vi "Laser-Repetition.vi"(2 "error in (no error)":errorcluster, 5 "VISA resource name":refnum<visa-resource-name>) -> (0 "error out":errorcluster, 1 "VISA resource name out":refnum<visa-resource-name>)   [LabVIEW 2013]
panel:
  # "uJ"
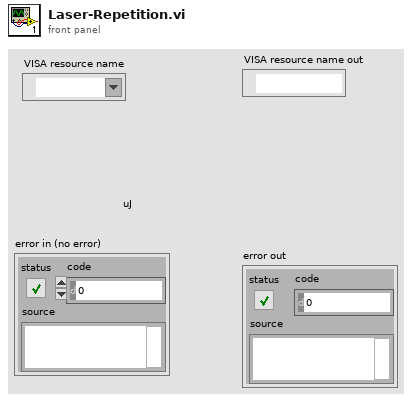
[diagram p1: front panel]
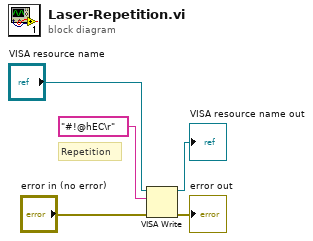
[diagram p0: block diagram]
diagram:
  # "Repetition"
  n1 = VISA Write(VISA resource name="VISA resource name", write buffer="#!@hEC\r", error in (no error)="error in (no error)") -> (VISA resource name out=→"VISA resource name out":refnum<visa-resource-name>, error out=→"error out":errorcluster)  [unwired: 1 out]
